vi "PRO_Check_ResistorV1.vi"(7 "ATP Check":bool, 8 "Results IN":T1(array[cluster])=[{"Fill"=0.0, "Drain"=0.0, "Status"=5, "Resistor"=101.0}, {"Fill"=0.0, "Drain"=7.375999999999938, "Status"=5, "Resistor"=201.0}, {"Fill"=7.28499999999994, "Drain"=6.925999999999948, "Status"=5, "Resistor"=301.0}, {"Fill"=6.834999999999949, "Drain"=6.489999999999958, "Status"=5, "Resistor"=401.0}, {"Fill"=6.375499999999959, "Drain"=6.035999999999967, "Status"=5, "Resistor"=501.0}, {"Fill"=5.924999999999969, "Drain"=5.584999999999977, "Status"=5, "Resistor"=601.0}, {"Fill"=5.484499999999978, "Drain"=5.125499999999986, "Status"=5, "Resistor"=701.0}, {"Fill"=5.024499999999988, "Drain"=4.675499999999996, "Status"=5, "Resistor"=801.0}, {"Fill"=4.570499999999997, "Drain"=4.235000000000006, "Status"=5, "Resistor"=901.0}, {"Fill"=4.124500000000007, "Drain"=3.784500000000014, "Status"=5, "Resistor"=1001.0}, {"Fill"=3.6750000000000167, "Drain"=3.335000000000024, "Status"=5, "Resistor"=1101.0}], 9 "Switched In":bool, 10 "Inputs":cluster{" Ohms":dbl, "Level OUt":dbl}={" Ohms"=101.0, "Level OUt"=8.030499999999925}, 11 "ChA Spec RNG In":T3={"Specs"=[8.5, 8.5, 7.425, 102.0, 98.0, 102.0, 98.0], "LUT Status"={"ChA/!ChB"=FALSE, "Drain/!Fill"=TRUE, "In Range?"=TRUE, "Switch Range?"=FALSE, "Measure R?"=TRUE, "Vaild R?"=TRUE, "Index(n)"=0, "Index(n)-1"=1, "Index Max"=13, "Index(n-1)"=0}}) -> (0 "results out":T1(array[cluster])=[{"Fill"=0.0, "Drain"=0.0, "Status"=5, "Resistor"=101.0}, {"Fill"=0.0, "Drain"=7.375999999999938, "Status"=5, "Resistor"=201.0}, {"Fill"=7.28499999999994, "Drain"=6.925999999999948, "Status"=5, "Resistor"=301.0}, {"Fill"=6.834999999999949, "Drain"=6.489999999999958, "Status"=5, "Resistor"=401.0}, {"Fill"=6.375499999999959, "Drain"=6.035999999999967, "Status"=5, "Resistor"=501.0}, {"Fill"=5.924999999999969, "Drain"=5.584999999999977, "Status"=5, "Resistor"=601.0}, {"Fill"=5.484499999999978, "Drain"=5.125499999999986, "Status"=5, "Resistor"=701.0}, {"Fill"=5.024499999999988, "Drain"=4.675499999999996, "Status"=5, "Resistor"=801.0}, {"Fill"=4.570499999999997, "Drain"=4.235000000000006, "Status"=5, "Resistor"=901.0}, {"Fill"=4.124500000000007, "Drain"=3.784500000000014, "Status"=5, "Resistor"=1001.0}, {"Fill"=3.6750000000000167, "Drain"=3.335000000000024, "Status"=5, "Resistor"=1101.0}], 1 "Level Out":T2={"Switched"=FALSE, "Level OUt"=8.030499999999925}, 2 "Err Num":i32, 3 "ChA Spec RNG Out":T3={"Specs"=[8.5, 8.5, 7.425, 102.0, 98.0, 102.0, 98.0], "LUT Status"={"ChA/!ChB"=FALSE, "Drain/!Fill"=TRUE, "In Range?"=TRUE, "Switch Range?"=FALSE, "Measure R?"=TRUE, "Vaild R?"=TRUE, "Index(n)"=0, "Index(n)-1"=1, "Index Max"=13, "Index(n-1)"=0}}, 5 "Switched Out":bool)   [LabVIEW 2024]
uses:
  Control Definitions/Def Spec RNG.ctl
  Control Definitions/Ded LUT_Status.ctl
  Control Definitions/Def_LevelSwitched.ctl
panel:
  out "Boolean 2":bool=TRUE
  out "Boolean":bool=TRUE
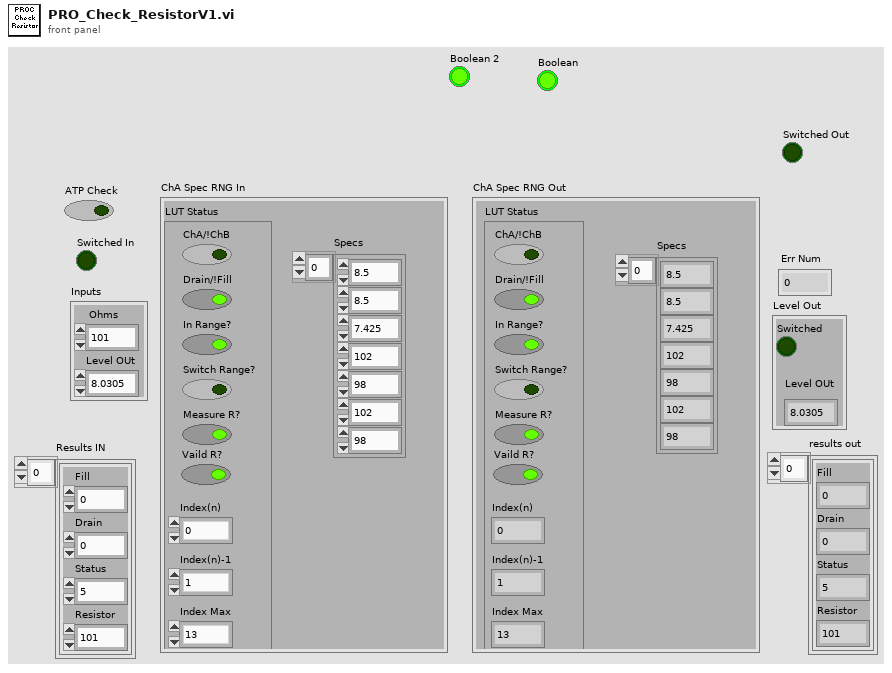
[diagram p1: front panel]
types:
  T1 = cluster{"Fill":dbl, "Drain":dbl, "Status":i16, "Resistor":dbl}[]
  T2 = typedef "Def_LevelSwitched.ctl" = cluster{"Switched":bool, "Level OUt":dbl}
  T3 = typedef "Def Spec RNG.ctl" = cluster{"Specs":dbl[], "LUT Status":T4}
  T4 = typedef "Ded LUT_Status.ctl" = cluster{"ChA/!ChB":bool, "Drain/!Fill":bool, "In Range?":bool, "Switch Range?":bool, "Measure R?":bool, "Vaild R?":bool, "Index(n)":i32, "Index(n)-1":i32, "Index Max":i32, "Index(n-1)":i32}
  T5 = cluster{"Fill":dbl, "Drain":dbl, "Status":i16, "Resistor":dbl}
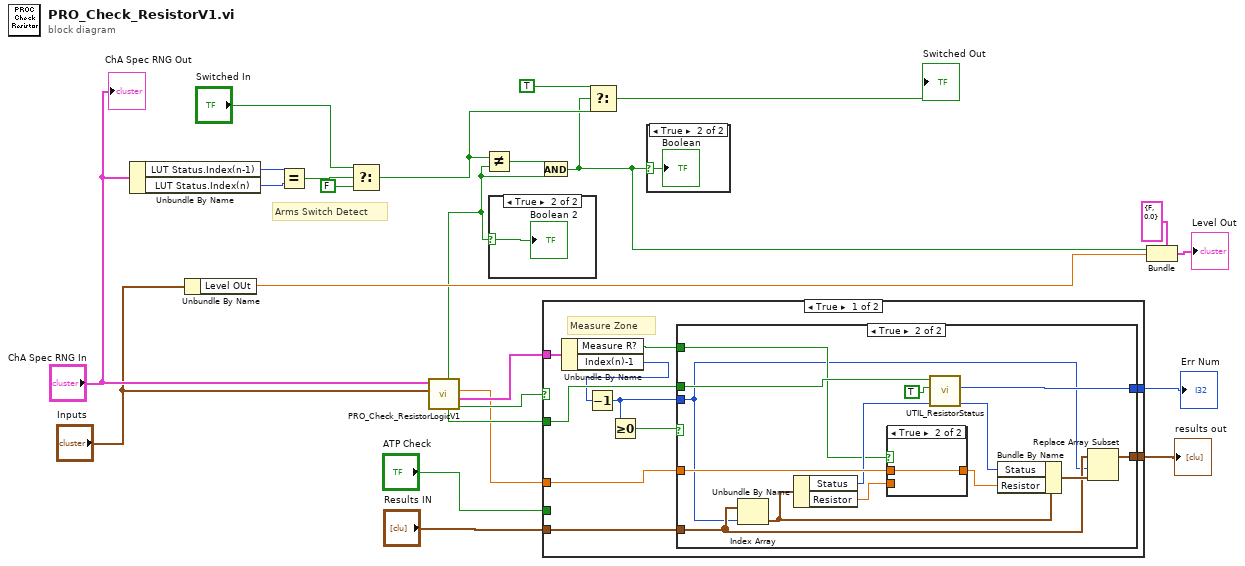
[diagram p0: block diagram]
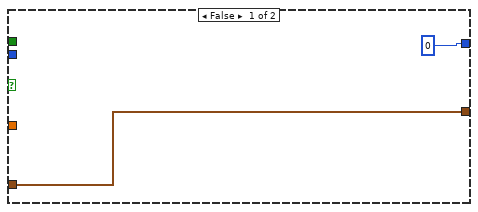
[diagram p4: hidden frame]
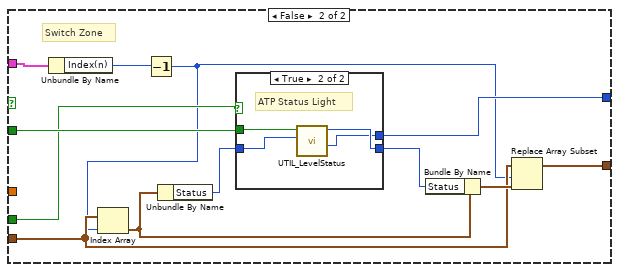
[diagram p6: hidden frame]
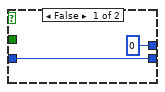
[diagram p7: hidden frame]
diagram:
  # "Arms Switch Detect"
  n1 = Unbundle By Name("ChA Spec RNG In") -> ("LUT Status.Index(n-1)"=w13:i32, "LUT Status.Index(n)"=w12:i32)
  n2 = Unbundle By Name("Inputs") -> ("Level OUt"=w10:dbl)
  n3 = Equal?(x=w13, y=w12) -> (x = y?=w5:bool)
  n4 = Select(t="Switched In", s=w5, f=FALSE) -> (s? t:f=w2:bool)
  n5 = call "PRO_Check_ResistorLogicV1.vi"("Inputs"="Inputs", "ChA Spec RNG In"="ChA Spec RNG In") -> ("Vaild R?"=w8:bool, "LUT Status"=w9:T4, "Resist Measured"=w7:dbl, "Resist in Spec"=w18:bool, "SwP Threshold?"=w6:bool)  [unwired: 4 in, 1 out]
  n6 = Not Equal?(x=w2, y=w6) -> (x != y?=w21:bool)
  n7 = case shown="True" w6 {
    selector: w6 -> [_ w25]
    frame False {
    }
    frame True {
      "Boolean 2" <- w25
    }
  }
  n8 = And(x=w21, y=w6) -> (x .and. y?=w1:bool)
  n9 = case shown="True" w8 {
    tunnel: w7 -> [w35 _]
    tunnel: [w34 w58] -> w24
    tunnel: w18 -> [w33 w60]
    tunnel: [w32 w64] -> w17
    tunnel: w9 -> [w31 w63]
    tunnel: "Results IN" -> [w29 w61]
    tunnel: "ATP Check" -> [_ w56]
    frame True {
      # "Measure Zone"
      n10 = Unbundle By Name(w31) -> ("Measure R?"=w30:bool, "Index(n)-1"=w28:i32)
      n11 = Decrement(x=w28) -> (x-1=w27:i32)
      n12 = Greater Or Equal To 0?(x=w27) -> (x >= 0?=w26:bool)
      n13 = case shown="True" w26 {
        tunnel: w35 -> [_ w51]
        tunnel: [0 ("Err Num") w48] -> w34
        tunnel: w33 -> [_ w47]
        tunnel: [w37 w42] -> w32
        tunnel: w30 -> [_ w41]
        tunnel: w29 -> [w37 w39]
        tunnel: w27 -> [_ w38]
        frame False {
        }
        frame True {
          n14 = Index Array(array=w39, index=w38) -> (element=w40:T5)
          n15 = Unbundle By Name(w40) -> ("Status"=w45:i16, "Resistor"=w49:dbl)
          n16 = case shown="True" w41 {
            tunnel: w51 -> [_ w53]
            tunnel: [w52 w53] -> w50
            tunnel: w49 -> [w52 _]
            frame False {
            }
            frame True {
            }
          }
          n17 = call "UTIL_ResistorStatus.vi"("Status in"=w45, "Measure?"=TRUE, "Good!Bad"=w47) -> ("Status out"=w44:u32, "Err Num"=w48:i32)  [unwired: 7 in]
          n18 = Bundle By Name(cluster=w40, "Status"=w44, "Resistor"=w50) -> (w43:T5)
          n19 = Replace Array Subset(array=w39, new element=w43, index=w38) -> (w42:T1)
        }
      }
    }
    frame False {
      # "Switch Zone"
      n20 = Unbundle By Name(w63) -> ("Index(n)"=w55:i32)
      n21 = Decrement(x=w55) -> (x-1=w54:i32)
      n22 = Index Array(array=w61, index=w54) -> (element=w62:T5)
      n23 = Unbundle By Name(w62) -> ("Status"=w59:i16)
      n24 = case shown="True" w56 {
        tunnel: [w67 w69] -> w57
        tunnel: w59 -> [w67 w70]
        tunnel: w60 -> [_ w71]
        tunnel: [u32 0 ("Err Num") w68] -> w58
        frame False {
        }
        frame True {
          # "ATP Status Light"
          n25 = call "UTIL_LevelStatus.vi"("Status In in"=w70, "Good!Bad"=w71) -> ("Err Num"=w68:u32, "Status In out"=w69:u32)  [unwired: 7 in, 1 out]
        }
      }
      n26 = Bundle By Name(cluster=w62, "Status"=w57) -> (w65:T5)
      n27 = Replace Array Subset(array=w61, new element=w65, index=w54) -> (w64:T1)
    }
  }
  "Err Num" <- w24
  "results out" <- w17
  n28 = Select(t=TRUE, s=w1, f=w2) -> (s? t:f=→"Switched Out":bool)
  n29 = case shown="True" w1 {
    selector: w1 -> [_ w72]
    frame False {
    }
    frame True {
      "Boolean" <- w72
    }
  }
  n30 = Bundle(cluster=cluster{bool, "Level OUt":dbl} {FALSE, "Level OUt"=0.0} ("output cluster"), w1, "Level OUt"=w10) -> (→"Level Out":cluster{bool, "Level OUt":dbl})
  "ChA Spec RNG Out" <- "ChA Spec RNG In"
